vi "Call Chain Trim Test.vi"() -> ()   [LabVIEW 2024]
uses:
  Formatters/Format String/Format String.lvclass
panel:
  out "shortened call chains":string
  in  "delimiter":string
  in  "call chain in":string[](array[string])
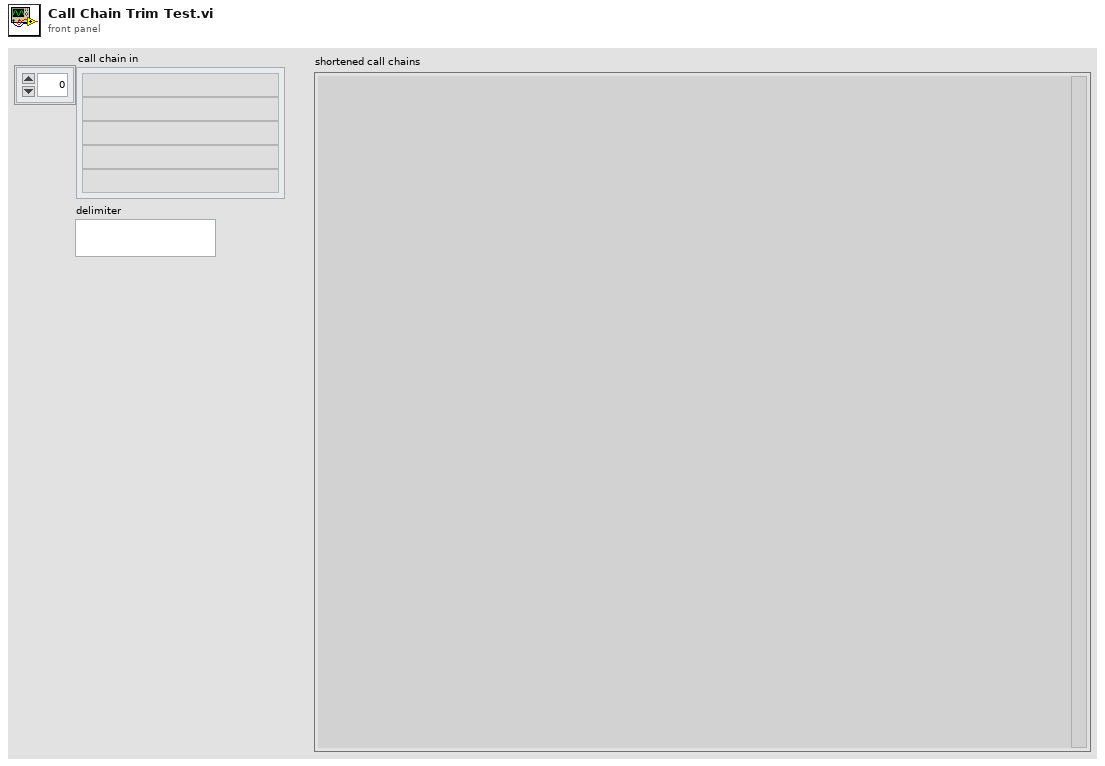
[diagram p1: front panel]
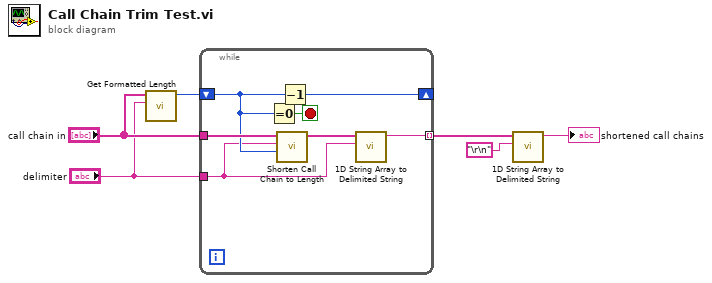
[diagram p0: block diagram]
diagram:
  n1 = call "Get Formatted Length.vi"("delimiter"="delimiter", "call chain"="call chain in") -> ("formatted length"=w1:u32)  [unwired: 9 in]
  n2 = while {
    tunnel: "call chain in" -> [w13]
    shift-right: [w10] -> _
    shift-left: w1 -> [w11]
    tunnel: "delimiter" -> [w7]
    tunnel: [w8] -> w4 mode=indexing
    stop <- w12 stop-if-true
    n3 = Equal To 0?(x=w11) -> (x = 0?=w12:bool)
    n4 = call "Shorten Call Chain to Length.vi"("desired length"=w11, "delimiter"=w7, "call chain in"=w13) -> ("call chain out"=w9:string[])  [unwired: 8 in]
    n5 = Decrement(x=w11) -> (x-1=w10:u32)
    n6 = call <vilib>:"1D String Array to Delimited String.vi"("delimiter"=w7, "string array"=w9) -> ("delimited string"=w8:string)  [unwired: 9 in]
  }
  n7 = call <vilib>:"1D String Array to Delimited String.vi"("delimiter"="\r\n", "string array"=w4) -> ("delimited string"=→"shortened call chains":string)  [unwired: 9 in]
